vi "MrClean.ProcCases.vi"(0 "i ref in":refnum<vi>, 1 "selector":string, 2 "Data":T1, 3 "call cluster":T2={"Object"="", "Selector"="", "CallType"=enum."synchronous", "Async Object"="", "Async Selector"="", "Data Descriptor"="", "Data"=[], "Error #"=0, "Expire"=0}, 5 "error in (no error)":errorcluster) -> (14 "i ref out":refnum<vi>, 17 "answer cluster":T2={"Object"="", "Selector"="", "CallType"=enum."synchronous", "Async Object"="", "Async Selector"="", "Data Descriptor"="", "Data"=[], "Error #"=0, "Expire"=0}, 19 "error out":errorcluster)   [LabVIEW 2014, in "MrClean.lvlib"]
doc: "This method is called by a process from within the default case in the event loop. The methods of a class that are linked to events will be called from THIS method. Add your code here."
uses:
  MrClean.lvlib
  CSCore/CSSystem/CoreDefs/CoreDefs.call_type.ctl
  CSCore/BaseProcess/BaseProcess.descriptor string definition.ctl
  CSCore/CSSystem/CoreDefs/CoreDefs.rawDataType.ctl
  CSCore/CSSystem/CoreLib/CoreLib.string 2 byte array.vi
  CSCore/CSSystem/CoreLib/CoreLib.byte array 2 double.vi
  CSCore/CSSystem/CoreLib/CoreLib.byte array 2 int.vi
  CSCore/BaseProcess/BaseProcess.lvlib
  CSCore/CSSystem/CoreLib/CoreLib.lvlib
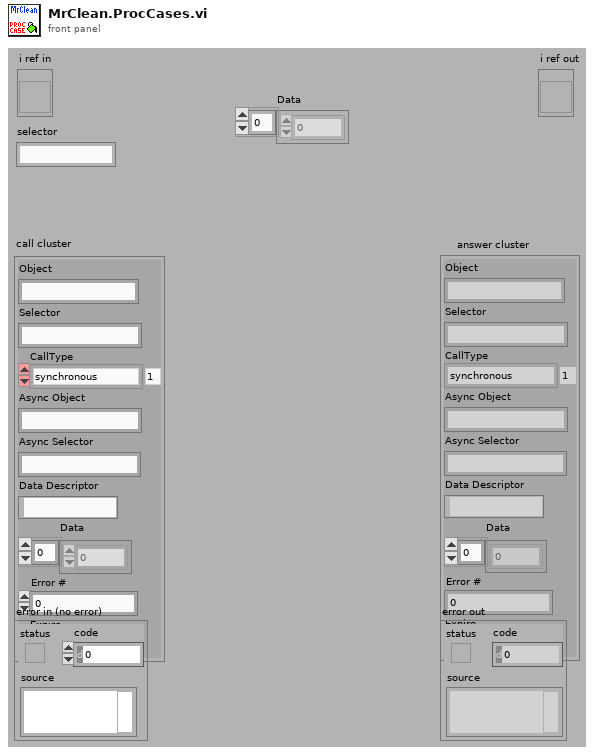
[diagram p1: front panel]
types:
  T1 = typedef "CoreDefs.rawDataType.ctl" = i8[]
  T2 = typedef "CoreDefs.call_type.ctl" = cluster{"Object":string, "Selector":string, "CallType":enum16{"simple", "synchronous", "asynchronous"}, "Async Object":string, "Async Selector":string, "Data Descriptor":T3, "Data":T1, "Error #":i32, "Expire":u32}
  T3 = typedef "BaseProcess.lvlib/BaseProcess.descriptor string definition.ctl" = string
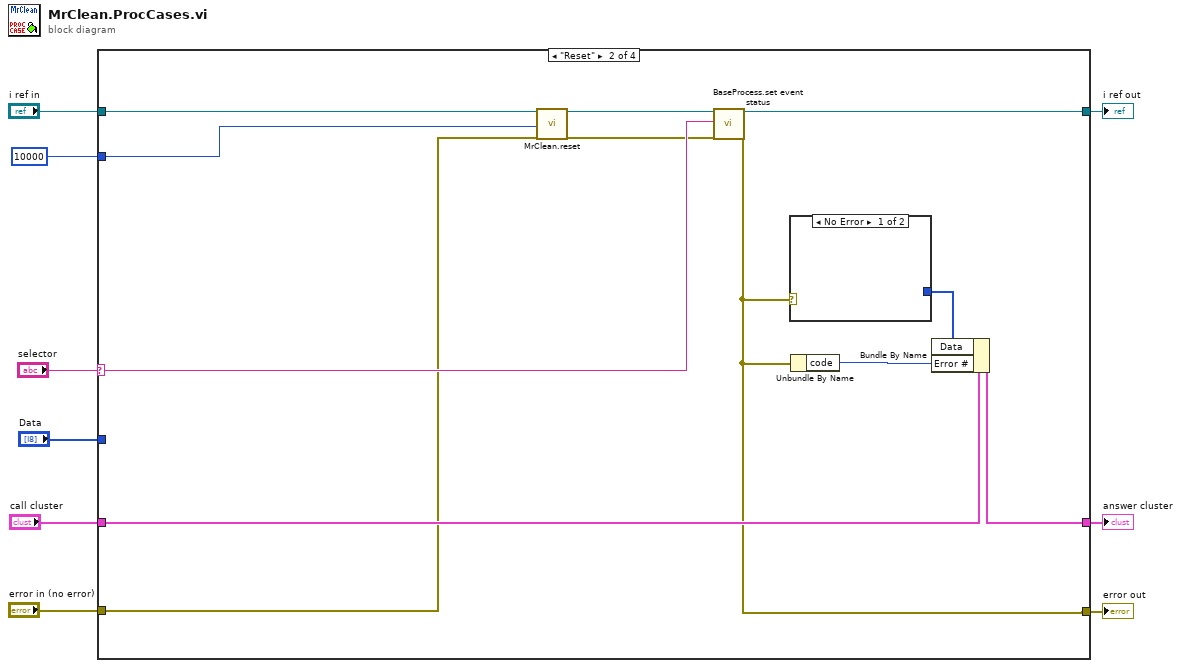
[diagram p0: block diagram]
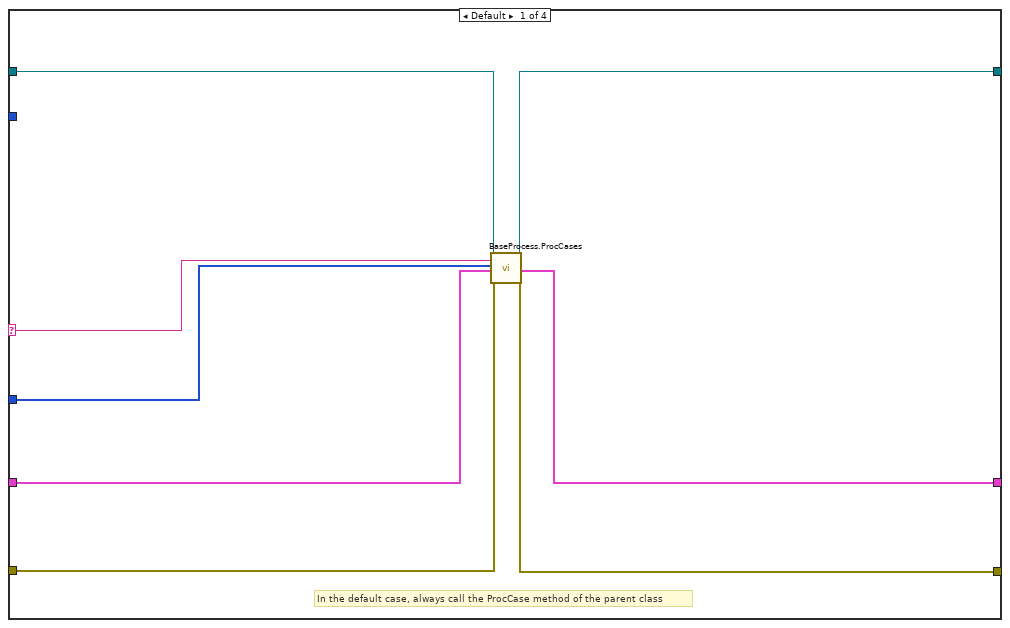
[diagram p2: hidden frame]
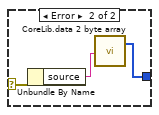
[diagram p3: hidden frame]
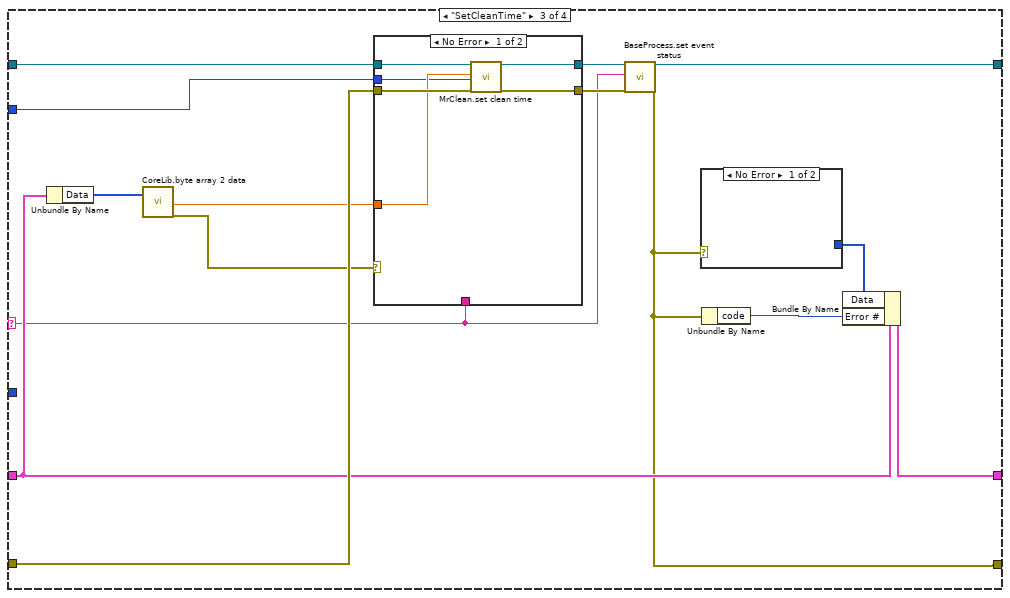
[diagram p4: hidden frame]
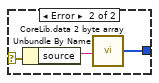
[diagram p5: hidden frame]
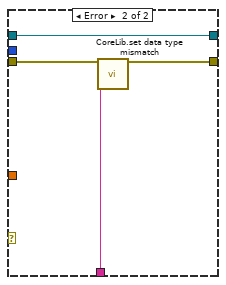
[diagram p6: hidden frame]
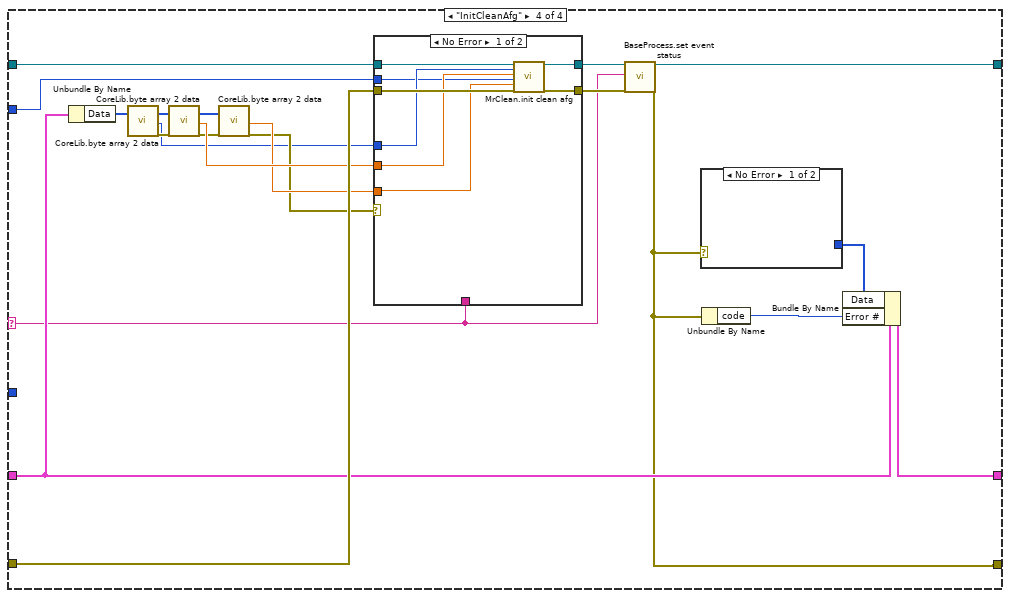
[diagram p7: hidden frame]
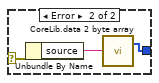
[diagram p8: hidden frame]
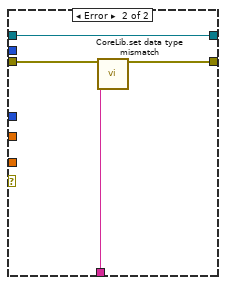
[diagram p9: hidden frame]
diagram:
  n1 = case shown="\"Reset\"" "selector" {
    selector: "selector" -> [w12 w25 w38 w72]
    tunnel: "i ref in" -> [w11 w23 w47 w81]
    tunnel: [w17 w24 w37 w71] -> w5
    tunnel: "call cluster" -> [w13 w28 w44 w78]
    tunnel: [w14 w27 w43 w77] -> w8
    tunnel: "error in (no error)" -> [w16 w21 w46 w80]
    tunnel: [w15 w26 w39 w73] -> w3
    tunnel: 10000 ("ms timeout (100)") -> [_ w19 w36 w70]
    tunnel: "Data" -> [w10 _ _ _]
    frame Default {
      # "In the default case, always call the ProcCase method of the parent class"
      n2 = call "BaseProcess.ProcCases.vi"("i ref in"=w11, "selector"=w12, "Data"=w10, "call cluster"=w13, "error in (no error)"=w16) -> ("i ref out"=w17:refnum<vi>, "answer cluster"=w14:T2, "error out"=w15:errorcluster)  [unwired: 12 in]
    }
    frame "Reset" {
      n3 = call "MrClean.reset.vi"("i ref in"=w23, "ms timeout (100)"=w19, "error in (no error)"=w21) -> ("i ref out"=w22:refnum<vi>, "error out"=w20:errorcluster)  [unwired: 14 in, 1 out]
      n4 = call "BaseProcess.set event status.vi"("i ref in"=w22, "EventStatus"=w25, "error in (no error)"=w20) -> ("i ref out"=w24:refnum<vi>, "error out"=w26:errorcluster)  [unwired: 14 in, 1 out]
      n5 = case shown="No Error" w26 {
        selector: w26 -> [_ w32]
        tunnel: [_ w30] -> w18
        frame No Error {
        }
        frame Error {
          n6 = Unbundle By Name(w32) -> ("source"=w31:string)
          n7 = call-poly "CoreLib.data 2 byte array.vi"("string"=w31) -> ("byteArray out"=w30:T1)  [unwired: 18 in]
        }
      }
      n8 = Unbundle By Name(w26) -> ("code"=w29:i32)
      n9 = Bundle By Name(cluster=w28, "Data"=w18, "Error #"=w29) -> (w27:T2)
    }
    frame "SetCleanTime" {
      n10 = Unbundle By Name(w44) -> ("Data"=w34:T1)
      n11 = call-poly "CoreLib.byte array 2 data.vi"("byteArray"=w34) -> ("d64"=w35:dbl, "error out"=w33:errorcluster)  [unwired: 16 in, 1 out]
      n12 = case shown="No Error" w33 {
        tunnel: [w55 w60] -> w41
        tunnel: w47 -> [w56 w60]
        tunnel: w46 -> [w53 w59]
        tunnel: [w54 w58] -> w40
        tunnel: w38 -> [_ w57]
        tunnel: w35 -> [w52 _]
        tunnel: w36 -> [w51 _]
        frame No Error {
          n13 = call "MrClean.set clean time.vi"("i ref in"=w56, "clean time [s]"=w52, "ms timeout (100)"=w51, "error in (no error)"=w53) -> ("i ref out"=w55:refnum<vi>, "error out"=w54:errorcluster)  [unwired: 13 in, 1 out]
        }
        frame Error {
          n14 = call "CoreLib.set data type mismatch.vi"("error in (no error)"=w59, "error source"=w57) -> ("error out"=w58:errorcluster)  [unwired: 17 in]
        }
      }
      n15 = call "BaseProcess.set event status.vi"("i ref in"=w41, "EventStatus"=w38, "error in (no error)"=w40) -> ("i ref out"=w37:refnum<vi>, "error out"=w39:errorcluster)  [unwired: 14 in, 1 out]
      n16 = case shown="No Error" w39 {
        selector: w39 -> [_ w50]
        tunnel: [_ w48] -> w42
        frame No Error {
        }
        frame Error {
          n17 = Unbundle By Name(w50) -> ("source"=w49:string)
          n18 = call-poly "CoreLib.data 2 byte array.vi"("string"=w49) -> ("byteArray out"=w48:T1)  [unwired: 18 in]
        }
      }
      n19 = Unbundle By Name(w39) -> ("code"=w45:i32)
      n20 = Bundle By Name(cluster=w44, "Data"=w42, "Error #"=w45) -> (w43:T2)
    }
    frame "InitCleanAfg" {
      n21 = Unbundle By Name(w78) -> ("Data"=w64:T1)
      n22 = call-poly "CoreLib.byte array 2 data.vi"("byteArray"=w64) -> ("byteArray out"=w62:T1, "i32"=w61:i32, "error out"=w63:errorcluster)  [unwired: 16 in]
      n23 = call-poly "CoreLib.byte array 2 data.vi"("byteArray"=w62, "error in (no error)"=w63) -> ("byteArray out"=w69:T1, "d64"=w68:dbl, "error out"=w66:errorcluster)  [unwired: 15 in]
      n24 = call-poly "CoreLib.byte array 2 data.vi"("byteArray"=w69, "error in (no error)"=w66) -> ("d64"=w67:dbl, "error out"=w65:errorcluster)  [unwired: 15 in, 1 out]
      n25 = case shown="No Error" w65 {
        tunnel: [w91 w96] -> w75
        tunnel: w81 -> [w92 w96]
        tunnel: w80 -> [w90 w95]
        tunnel: [w89 w94] -> w74
        tunnel: w68 -> [w87 _]
        tunnel: w72 -> [_ w93]
        tunnel: w61 -> [w88 _]
        tunnel: w67 -> [w86 _]
        tunnel: w70 -> [w85 _]
        frame No Error {
          n26 = call "MrClean.init clean afg.vi"("i ref in"=w92, "CleanAfg"=w88, "amplitude [V]"=w87, "ms timeout (100)"=w85, "frequency [Hz]"=w86, "error in (no error)"=w90) -> ("i ref out"=w91:refnum<vi>, "error out"=w89:errorcluster)  [unwired: 11 in, 1 out]
        }
        frame Error {
          n27 = call "CoreLib.set data type mismatch.vi"("error in (no error)"=w95, "error source"=w93) -> ("error out"=w94:errorcluster)  [unwired: 17 in]
        }
      }
      n28 = call "BaseProcess.set event status.vi"("i ref in"=w75, "EventStatus"=w72, "error in (no error)"=w74) -> ("i ref out"=w71:refnum<vi>, "error out"=w73:errorcluster)  [unwired: 14 in, 1 out]
      n29 = case shown="No Error" w73 {
        selector: w73 -> [_ w84]
        tunnel: [_ w82] -> w76
        frame No Error {
        }
        frame Error {
          n30 = Unbundle By Name(w84) -> ("source"=w83:string)
          n31 = call-poly "CoreLib.data 2 byte array.vi"("string"=w83) -> ("byteArray out"=w82:T1)  [unwired: 18 in]
        }
      }
      n32 = Unbundle By Name(w73) -> ("code"=w79:i32)
      n33 = Bundle By Name(cluster=w78, "Data"=w76, "Error #"=w79) -> (w77:T2)
    }
  }
  "answer cluster" <- w8
  "i ref out" <- w5
  "error out" <- w3
